vi "PXI-Enumerate Channels on Device.vi"(0 "ActiveDev":tag, 11 "error in (no error)":errorcluster) -> (4 "AO":string[](array[string]), 8 "AI":string[](array[string]), 15 "error out":errorcluster)   [LabVIEW 2015]
uses:
  <resource>/objmgr/daqmx.rc
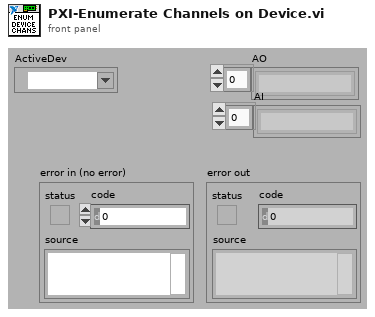
[diagram p1: front panel]
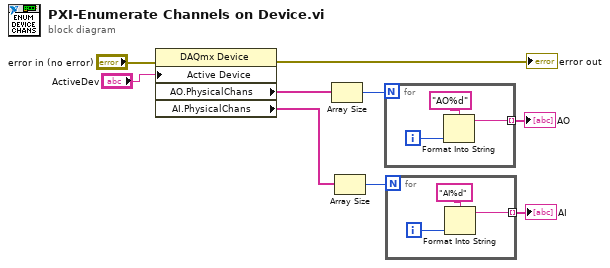
[diagram p0: block diagram]
diagram:
  n1 = property class="DAQmx Device"(error in="error in (no error)", "Active Device"="ActiveDev") -> (error out=→"error out":errorcluster, "AO.PhysicalChans"=w7:tag[], "AI.PhysicalChans"=w6:tag[])  [unwired: 1 in, 1 out]
  n2 = Array Size(array=w7) -> (size(s)=w4:i32)
  n3 = Array Size(array=w6) -> (size(s)=w2:i32)
  n4 = for {
    N: w4 -> [_]
    tunnel: [w10] -> w3 mode=indexing
    i -> [w11]
    n5 = Format Into String(format string="AO%d", w11) -> (resulting string=w10:string)  [unwired: 2 in, 1 out]
  }
  "AO" <- w3
  n6 = for {
    N: w2 -> [_]
    tunnel: [w13] -> w1 mode=indexing
    i -> [w14]
    n7 = Format Into String(format string="AI%d", w14) -> (resulting string=w13:string)  [unwired: 2 in, 1 out]
  }
  "AI" <- w1
